vi "ConfigureSimulatedHardware.vi"(8 "error in (no error)":errorcluster, 11 "configuration":T1 {"HighPassFilterState"."Filter State" format="%.2f"; "HighPassFilterState"."IIR Filter Cluster"."Forward Coefficients" format="%.2f"; "HighPassFilterState"."IIR Filter Cluster"."Reverse Coefficients" format="%.2f"; "FixedSizeX32"."InputConfig" items=["AC Coupled", "DC Coupled", "IEPE AC Coupled"]}) -> (0 "error out":errorcluster, 3 "configuration out":T1={"Acq"=FALSE, "NumberOfModules"=0, "Dynamic FPGA VI Ref"=refnum, "KeyphasorX3"=[], "FixedSizeX32"={"EnabledChannels"=[], "Sensitivity"=[], "InputConfig"=[]}, "SamplingInfo"={"Number of Channels"=4, "Sampling Rate"=4.0, "Channels"=[], "Units"=[], "Offsets"=[]}, "Normal Mode Sample Rate"=0.0, "BlockSize (sec)"=0.0, "Samples To Read (per chan)"=0, "RunningAcquisitionLength"=0.0, "Settling Time"=0.0, "Waveform Groups"=[], "Acquisition Block Number"=0, "Device Name"="", "ValidConfig"=FALSE, "Last Dynamic Module"="", "HighPassFilterState"=[], "Low Frequency Cutoff"=[], "BurstMode"={"Acquisition Time"=0.0, "Sample Rate"=0.0, "Collection Reason"=""}} {"HighPassFilterState"."Filter State" format="%.2f"; "HighPassFilterState"."IIR Filter Cluster"."Forward Coefficients" format="%.2f"; "HighPassFilterState"."IIR Filter Cluster"."Reverse Coefficients" format="%.2f"; "FixedSizeX32"."InputConfig" items=["AC Coupled", "DC Coupled", "IEPE AC Coupled"]})   [LabVIEW 2017, in "CmsAcquisition.lvlib"]
uses:
  <vilib>/addons/InsightCM/Devices/Shared/Cms/CmsAcquisition/CmsAcquisition.lvlib
  <vilib>/addons/InsightCM/Devices/Shared/Cms/CmsAcquisition/controls/Configuration.ctl
  <vilib>/addons/InsightCM/Devices/Shared/Cms/CmsAcquisition/controls/TachometerConfig.ctl
  <vilib>/addons/InsightCM/Devices/Shared/Cms/CmsAcquisition/controls/FixedSizeArrays.ctl
  <vilib>/LabVIEW Targets/FPGA/cRIO/shared/nicrio_ModuleControls/nicrio_cRIO-9232_ConfigModeRing.ctl
  <vilib>/addons/InsightCM/Devices/Shared/Cms/cRIOWfmAcq/subVIs/RIO Wfm Cust Ctrls/rwfm_SamplingInfo.ctl
  <vilib>/addons/InsightCM/Devices/Shared/Cms/CmsAcquisition/controls/Group.ctl
  <vilib>/addons/InsightCM/Devices/Shared/Cms/CmsAcquisition/controls/Channel.ctl
  <vilib>/addons/InsightCM/Utilities/Analysis/Vibration/controls/HighPassFilterState.ctl
  <vilib>/addons/InsightCM/Devices/Shared/Cms/CmsAcquisition/controls/BurstMode.ctl
  <vilib>/addons/InsightCM/Devices/Shared/Cms/CmsAcquisition/controls/AcqSimulated_SignalConfig.ctl
  <vilib>/addons/InsightCM/Devices/Shared/Cms/CmsAcquisition/controls/AcqSimulated_Channels.ctl
  <vilib>/addons/InsightCM/Devices/Shared/Cms/CmsAcquisition/subVIs/SimulatedConfigRefGlobal.vi
  <vilib>/addons/InsightCM/Devices/Shared/Cms/cRIOWfmAcq/cRIOWfmLib.lvlib
  <vilib>/addons/InsightCM/Utilities/Analysis/Vibration/VibrationAnalysisFunctions.lvlib
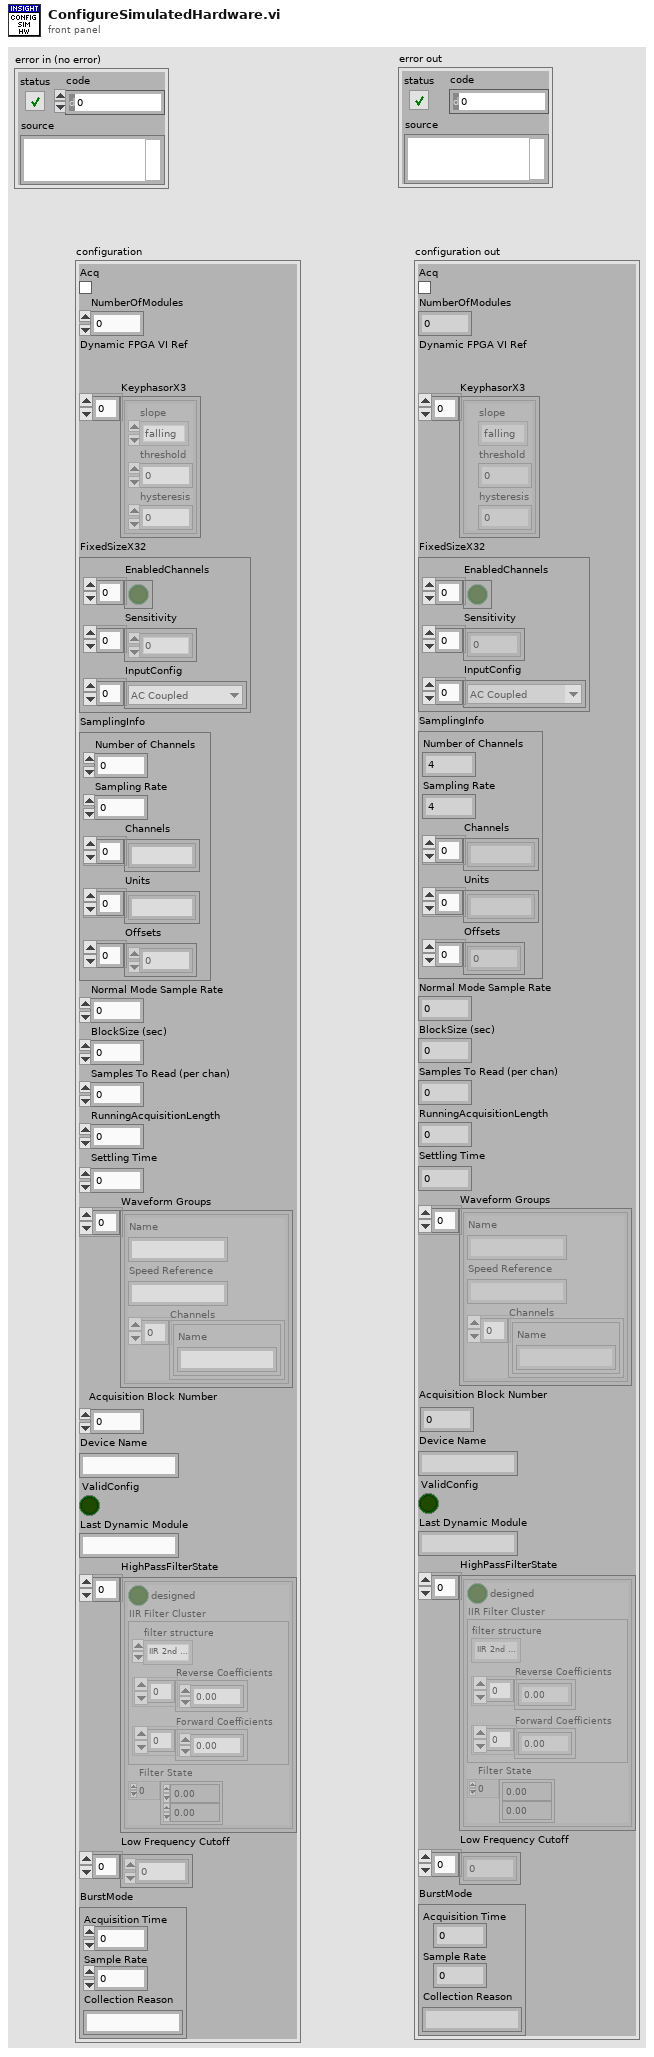
[diagram p1: front panel]
types:
  T1 = typedef "CmsAcquisition.lvlib/Configuration.ctl" = cluster{"Acq":bool, "NumberOfModules":i16, "Dynamic FPGA VI Ref":refnum<k20>, "KeyphasorX3":T2[], "FixedSizeX32":T3, "SamplingInfo":T5, "Normal Mode Sample Rate":dbl, "BlockSize (sec)":dbl, "Samples To Read (per chan)":i32, "RunningAcquisitionLength":dbl, "Settling Time":dbl, "Waveform Groups":T6[], "Acquisition Block Number":i32, "Device Name":string, "ValidConfig":bool, "Last Dynamic Module":string, "HighPassFilterState":T8[], "Low Frequency Cutoff":dbl[], "BurstMode":T9}
  T2 = typedef "CmsAcquisition.lvlib/TachometerConfig.ctl" = cluster{"slope":enum16{"falling", "rising"}, "threshold":dbl, "hysteresis":dbl}
  T3 = typedef "CmsAcquisition.lvlib/FixedSizeArrays.ctl" = cluster{"EnabledChannels":bool[], "Sensitivity":dbl[], "InputConfig":T4[]}
  T4 = typedef "nicrio_cRIO-9232_ConfigModeRing.ctl" = u8
  T5 = typedef "cRIOWfmLib.lvlib/rwfm_SamplingInfo.ctl" = cluster{"Number of Channels":i32, "Sampling Rate":dbl, "Channels":string[], "Units":string[], "Offsets":sgl[]}
  T6 = typedef "CmsAcquisition.lvlib/Group.ctl" = cluster{"Name":string, "Speed Reference":string, "Channels":T7[]}
  T7 = typedef "CmsAcquisition.lvlib/Channel.ctl" = cluster{"Name":string}
  T8 = typedef "VibrationAnalysisFunctions.lvlib/HighPassFilterState.ctl" = cluster{"designed":bool, "IIR Filter Cluster":cluster{"filter structure":enum32{"IIR 2nd Order", "IIR 4th Order"}, "Reverse Coefficients":dbl[], "Forward Coefficients":dbl[]}, "Filter State":dbl[]}
  T9 = typedef "CmsAcquisition.lvlib/BurstMode.ctl" = cluster{"Acquisition Time":dbl, "Sample Rate":dbl, "Collection Reason":string}
  T10 = enum16{"None", "Pk_PkPK", "N Rule", "Z Rule", "U Rule", "Line Noise", "Low Signal", "Ski Slope", "Envelope Test"}
  T11 = cluster{"order.":i32, "mag (rms)":i32, "phase (°)":dbl}
  T12 = typedef "CmsAcquisition.lvlib/AcqSimulated_SignalConfig.ctl" = cluster{"SimChannels":T13, "DutyCycle (%)":dbl, "Add Noise?":bool, "NoiseAmplitude":dbl, "Offset":dbl, "SamplingInfo":cluster{"Fs":dbl, "#s":dbl}, "TachMode1-Ch0":bool, "Offsets":dbl[]}
  T13 = typedef "CmsAcquisition.lvlib/AcqSimulated_Channels.ctl" = cluster{"Name":string[], "Vibration":cluster{"order.":dbl, "mag (rms)":dbl, "phase (°)":dbl}[][]}
  T14 = typedef "CmsAcquisition.lvlib/AcqSimulated_ConfigRefs.ctl" = cluster{"SignalConfigReference":refnum<vi>, "TachometerConfigReference":refnum<vi>}
  T15 = typedef "FpgaAcquisition923x.lvlib/AcqSimulated_SignalConfig.ctl" = cluster{"SimChannels":T16, "DutyCycle (%)":dbl, "Add Noise?":bool, "NoiseAmplitude":dbl, "Offset":dbl, "SamplingInfo":cluster{"Fs":dbl, "#s":dbl}, "TachMode1-Ch0":bool, "Offsets":dbl[]}
  T16 = typedef "FpgaAcquisition923x.lvlib/AcqSimulated_Channels.ctl" = cluster{"Name":string[], "Vibration":cluster{"order.":dbl, "mag (rms)":dbl, "phase (°)":dbl}[][]}
  T17 = cluster{"order.":dbl, "mag (rms)":dbl, "phase (°)":dbl}[][]
  T18 = cluster{"order.":i32, "mag (rms)":i32, "phase (°)":dbl}[][]
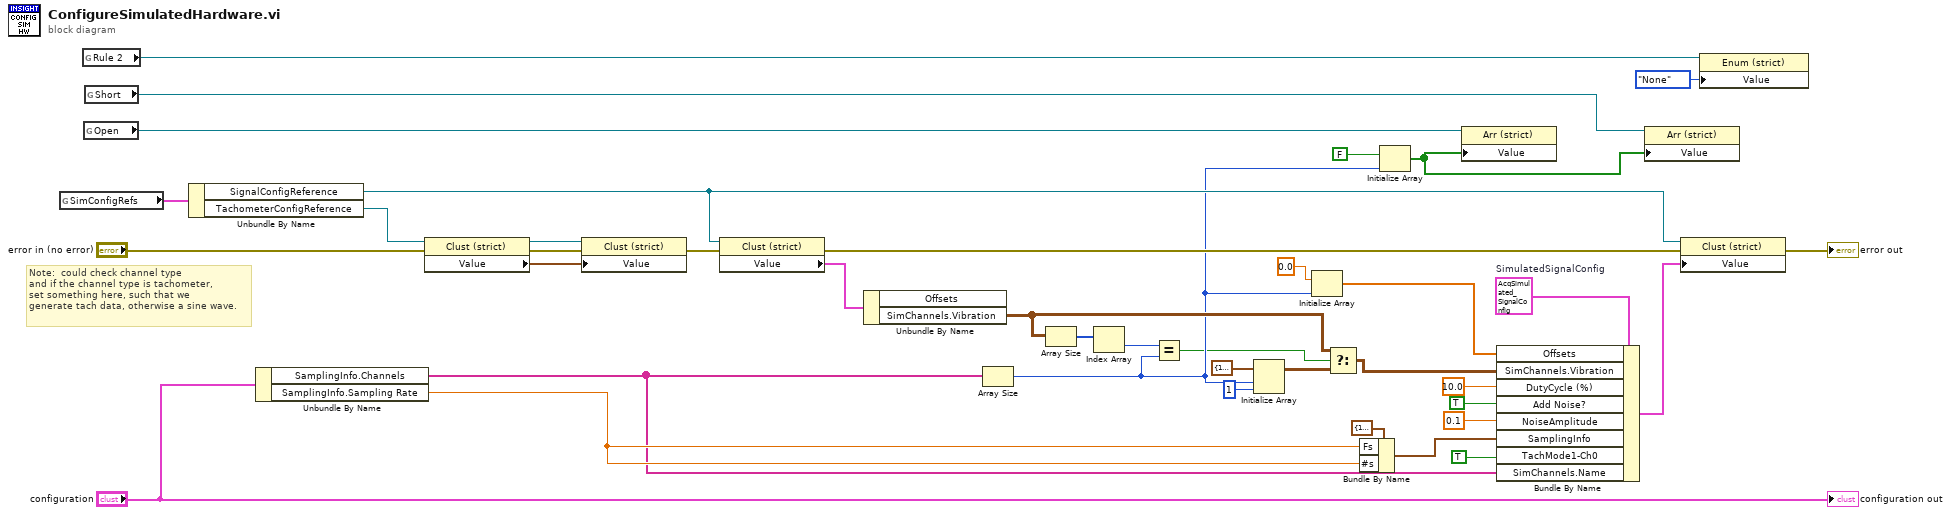
[diagram p0: block diagram]
diagram:
  w35 = T12 {"SimChannels"={"Name"=[], "Vibration"=[]}, "DutyCycle (%)"=10.0, "Add Noise?"=TRUE, "NoiseAmplitude"=0.1, "Offset"=0.0, "SamplingInfo"={"Fs"=1000.0, "#s"=1000.0}, "TachMode1-Ch0"=FALSE, "Offsets"=[]}  # SimulatedSignalConfig
  # "Note:  could check channel type\nand if the channel type is tachometer,\nset something here, such that we\ngenerate tach data, otherwise a sine wave."
  n1 = global read "SimulatedConfigRefGlobal.vi" "SimConfigRefs"() -> (w31:T14)
  n2 = global read "SimulatedConfigRefGlobal.vi" "Rule 2"() -> (w23:refnum<vi>)
  n3 = global read "SimulatedConfigRefGlobal.vi" "Open"() -> (w27:refnum<vi>)
  n4 = global read "SimulatedConfigRefGlobal.vi" "Short"() -> (w25:refnum<vi>)
  n5 = Unbundle By Name(w31) -> ("SignalConfigReference"=w17:refnum<vi>, "TachometerConfigReference"=w5:refnum<vi>)
  n6 = Unbundle By Name("configuration") -> ("SamplingInfo.Channels"=w14:string[], "SamplingInfo.Sampling Rate"=w29:dbl)
  n7 = property class="Clust (strict)"(reference=w5, error in="error in (no error)") -> (reference out=w4:refnum<vi>, error out=w3:errorcluster, "Value"=w1:cluster{"RPM":sgl})
  n8 = property class="Clust (strict)"(reference=w4, error in=w3, "Value"=w1) -> (error out=w18:errorcluster)  [unwired: 1 out]
  n9 = property class="Clust (strict)"(reference=w17, error in=w18) -> (error out=w16:errorcluster, "Value"=w15:T15)  [unwired: 1 out]
  n10 = Unbundle By Name(w15) -> ("SimChannels.Vibration"=w12:T17)  [unwired: 1 out]
  n11 = Array Size(array=w14) -> (size(s)=w7:i32)
  n12 = Array Size(array=w12) -> (size(s)=w9:i32[])
  n13 = Index Array(array=w9) -> (element=w8:i32)  [unwired: 1 in]
  n14 = Equal?(x=w8, y=w7) -> (x = y?=w6:bool)
  n15 = Initialize Array(T11 {"order."=1, "mag (rms)"=1, "phase (°)"=0.0} ("Harmonic"), w7, 1 ("dimension size")) -> (w11:T18)
  n16 = Initialize Array(0.0 ("Offset"), w7) -> (w13:dbl[])
  n17 = Select(t=w12, s=w6, f=w11) -> (s? t:f=w10:T17)
  n18 = Bundle By Name(cluster=cluster{"Fs":dbl, "#s":dbl} {"Fs"=1000.0, "#s"=1000.0} ("SamplingInfo"), "Fs"=w29, "#s"=w29) -> (w28:cluster{"Fs":dbl, "#s":dbl})
  n19 = Initialize Array(FALSE ("Add Noise?"), w7) -> (w24:bool[])
  n20 = property class="Arr (strict)"(reference=w27, "Value"=w24) -> ()  [unwired: 1 in, 2 out]
  n21 = Bundle By Name(cluster=w35, "Offsets"=w13, "SimChannels.Vibration"=w10, "DutyCycle (%)"=10.0, "Add Noise?"=TRUE, "NoiseAmplitude"=0.1, "SamplingInfo"=w28, "TachMode1-Ch0"=TRUE, "SimChannels.Name"=w14) -> (w21:T12)
  n22 = property class="Arr (strict)"(reference=w25, "Value"=w24) -> ()  [unwired: 1 in, 2 out]
  n23 = property class="Clust (strict)"(reference=w17, error in=w16, "Value"=w21) -> (error out=→"error out":errorcluster)  [unwired: 1 out]
  n24 = property class="Enum (strict)"(reference=w23, "Value"=T10."None") -> ()  [unwired: 1 in, 2 out]
  "configuration out" <- "configuration"
